vi "Read Configuration String.vi"(8 "error in (no error)":errorcluster, 10 "Config string":string, 11 "TDCManager":T1) -> (0 "error out":errorcluster, 2 "Success?":bool, 3 "TDCManager":T1)   [LabVIEW 2016, in "HPTDC Driver Library.lvlib"]
uses:
  HPTDC Driver Library.lvlib
  Typedefs/TDCManager.ctl
  C:/Users/CRT Controller/CRTC Labview Application/Source/HPTDC Driver Library Folder/Library files/hptdc_net4_3.7.0_x64.dll
  hptdc_net4_3.7.0_x64.dll
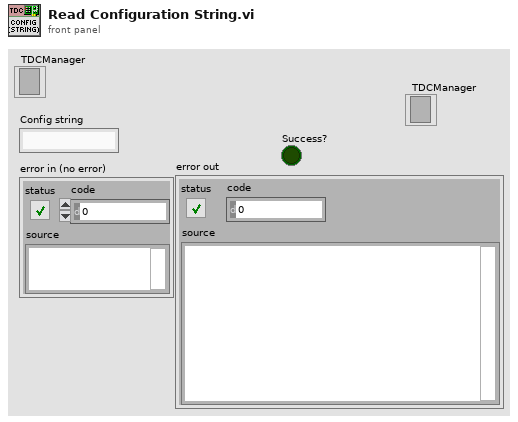
[diagram p1: front panel]
types:
  T1 = typedef "HPTDC Driver Library.lvlib/TDCManager.ctl" = refnum<k24>
  T2 = typedef "Semaphore RefNum" = refnum<k1>
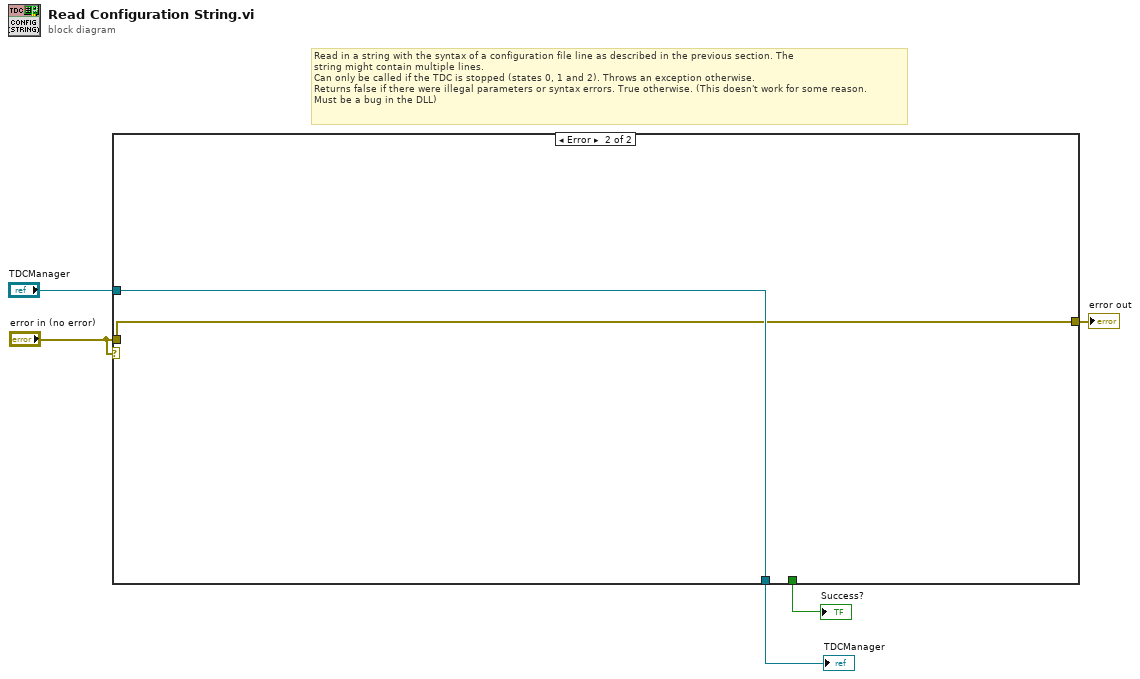
[diagram p0: block diagram]
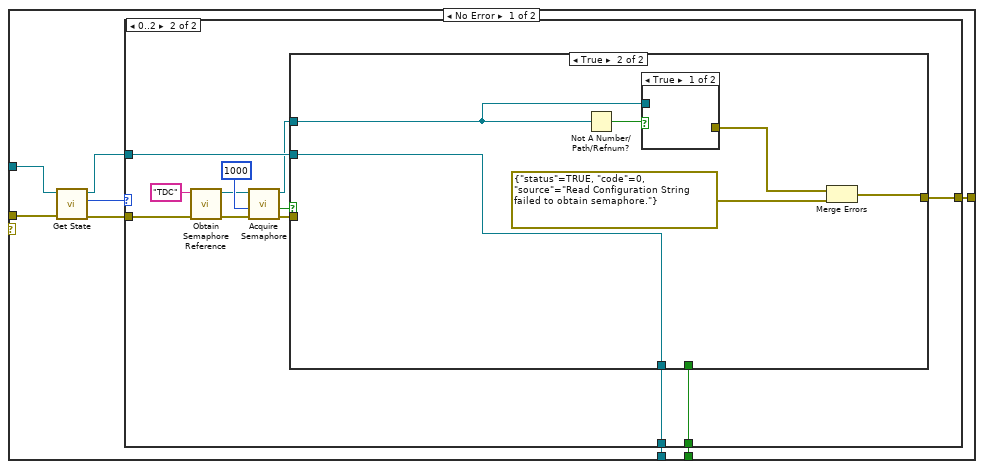
[diagram p2: hidden frame]
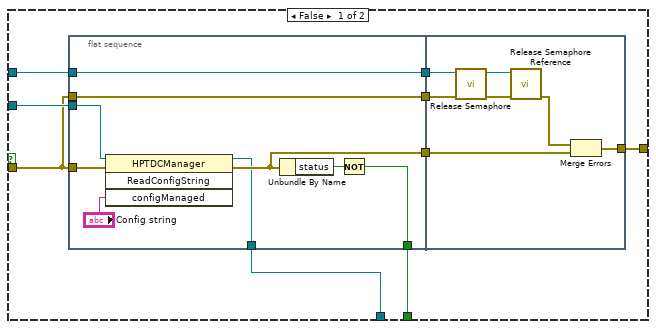
[diagram p4: hidden frame]
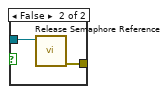
[diagram p5: hidden frame]
diagram:
  # "Read in a string with the syntax of a configuration file line as described in the previous section. The\nstring might contain multiple lines.\nCan only be called if the TDC is stopped (states 0, 1 and 2). Throws an exception otherwise.\nReturns false if there were illegal parameters or syntax errors. True otherwise. (This doesn't work for some reason.\nMust be a bug in the DLL)"
  n1 = case shown="Error" "error in (no error)" {
    tunnel: "TDCManager" -> [w13 w62]
    tunnel: "error in (no error)" -> [w12 w61]
    tunnel: [w8 w61] -> w4
    tunnel: [w7 _] -> w3
    tunnel: [w6 w62] -> w2
    frame No Error {
      n2 = call "Get State.vi"("error in"=w12, "TDCManager"=w13) -> ("error out"=w9:errorcluster, "State"=w11:i32, "TDCManager"=w10:T1)  [unwired: 6 in, 1 out]
      n3 = case shown="0..2" w11 {
        tunnel: w9 -> [w15 w22]
        tunnel: w10 -> [w14 w27]
        tunnel: [_ w18] -> w7
        tunnel: [w14 w17] -> w6
        tunnel: [w15 w16] -> w8
        frame Default {
        }
        frame 0..2 {
          n4 = call <vilib>:"Obtain Semaphore Reference.vi"("error in (no error)"=w22, "name (unnamed)"="TDC") -> ("error out"=w24:errorcluster, "semaphore"=w25:T2)  [unwired: 3 in, 1 out]
          n5 = call <vilib>:"Acquire Semaphore.vi"("error in (no error)"=w24, "ms timeout (-1)"=1000, "semaphore"=w25) -> ("error out"=w20:errorcluster, "timed out"=w21:bool, "semaphore out"=w19:T2)  [unwired: 2 in]
          n6 = case shown="True" w21 {
            tunnel: w27 -> [w36 w54]
            tunnel: w20 -> [w33 _]
            tunnel: w19 -> [w31 w53]
            tunnel: [w30 _] -> w18
            tunnel: [w29 w54] -> w17
            tunnel: [w28 w55] -> w16
            frame False {
              n7 = flat-sequence {
                tunnel: w33 -> [w45]
                tunnel: w36 -> [w44]
                tunnel: [w43] -> w35
                tunnel: w33 -> [w40]
                tunnel: [w40] -> w34
                tunnel: [w39] -> w32
                tunnel: w31 -> [w39]
                tunnel: [w37] -> w30
                tunnel: [w38] -> w29
                tunnel: w35 -> [w52]
                tunnel: w34 -> [w49]
                tunnel: w32 -> [w47]
                tunnel: [w46] -> w28
                frame #0 {
                  n8 = invoke class="HPTDCManager" method="ReadConfigString"(reference=w44, error in=w45, "configManaged"="Config string") -> (reference out=w38:T1, error out=w43:errorcluster)  [unwired: 1 in, 2 out]
                  n9 = Unbundle By Name(w43) -> ("status"=w42:bool)
                  n10 = Not(x=w42) -> (.not. x?=w37:bool)
                }
                frame #1 {
                  n11 = call <vilib>:"Release Semaphore.vi"("error in (no error)"=w49, "semaphore"=w47) -> ("error out"=w50:errorcluster, "semaphore out"=w51:T2)  [unwired: 4 in]
                  n12 = call <vilib>:"Release Semaphore Reference.vi"("error in (no error)"=w50, "semaphore"=w51) -> ("error out"=w48:errorcluster)  [unwired: 8 in, 1 out]
                  n13 = Merge Errors(w48, w52) -> (w46:errorcluster)
                }
              }
            }
            frame True {
              n14 = Not A Number/Path/Refnum?(number/path/refnum=w53) -> (NaN/Path/Refnum?=w58:bool)
              n15 = case shown="True" w58 {
                tunnel: [_ w60] -> w57
                tunnel: w53 -> [_ w59]
                frame True {
                }
                frame False {
                  n16 = call <vilib>:"Release Semaphore Reference.vi"("semaphore"=w59) -> ("error out"=w60:errorcluster)  [unwired: 9 in, 1 out]
                }
              }
              n17 = Merge Errors(w57, errorcluster {"status"=TRUE, "code"=0, "source"="Read Configuration String failed to obtain semaphore."} ("error out")) -> (w55:errorcluster)
            }
          }
        }
      }
    }
    frame Error {
    }
  }
  "error out" <- w4
  "Success?" <- w3
  "TDCManager" <- w2
